vi "Register Sessions Impl.vi"(8 "error in":errorcluster, 11 "data in":T1) -> (0 "error out":errorcluster, 3 "data out":T1)   [LabVIEW 2020, in "MeasurementLink Session Management.lvlib" / "Session Reservation.lvclass"]
uses:
  Session Reservation.lvclass
  Data.ctl
  Connection Map/Connection Map.lvclass
  IState/IState.lvclass
  Session and Driver Info.ctl
  MeasurementLink Instrument/IInstrument/IInstrument.lvclass
  MeasurementLink Session Management Client/RPC Messages/ni_measurementlink_sessionmanagement_v1_SessionInformation.ctl
  MeasurementLink Session Management Client/RPC Messages/nidevice_grpc_Session.ctl
  MeasurementLink Session Management Client/RPC Messages/ni_measurementlink_sessionmanagement_v1_ChannelMapping.ctl
  MeasurementLink Session Management Client/RPC Messages/ni_measurementlink_PinMapContext.ctl
  MeasurementLink gRPC Utilities/gRPC Client Pool/FGV Action.ctl
  MeasurementLink Session Management Client/RPC Messages/ni_measurementlink_sessionmanagement_v1_RegisterSessionsRequest.ctl
  MeasurementLink gRPC Utilities/gRPC Client Pool/gRPC Client Pool.lvclass
  MeasurementLink Session Management Client/MeasurementLink Session Management Client.lvlib
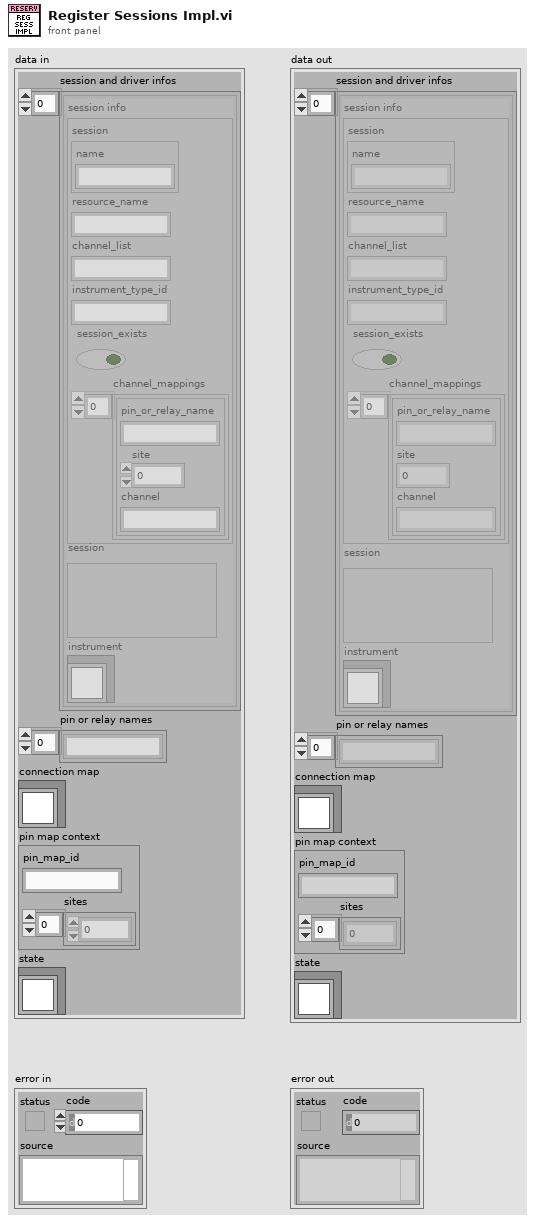
[diagram p1: front panel]
types:
  T1 = typedef "MeasurementLink Session Management.lvlib/Session Reservation.lvclass/Data.ctl" = cluster{"session and driver infos":T2[], "pin or relay names":string[], "connection map":refnum<class "Connection Map.lvclass">, "pin map context":T6, "state":refnum<class "IState.lvclass">}
  T2 = typedef "MeasurementLink Session Management.lvlib/Session Reservation.lvclass/Session and Driver Info.ctl" = cluster{"session info":T3, "session":variant, "instrument":refnum<class "IInstrument.lvclass">}
  T3 = typedef "MeasurementLink Session Management Client.lvlib/ni_measurementlink_sessionmanagement_v1_SessionInformation.ctl" = cluster{"session":T4, "resource_name":string, "channel_list":string, "instrument_type_id":string, "session_exists":bool, "channel_mappings":T5[]}
  T4 = typedef "MeasurementLink Session Management Client.lvlib/nidevice_grpc_Session.ctl" = cluster{"name":string}
  T5 = typedef "MeasurementLink Session Management Client.lvlib/ni_measurementlink_sessionmanagement_v1_ChannelMapping.ctl" = cluster{"pin_or_relay_name":string, "site":i32, "channel":string}
  T6 = typedef "MeasurementLink Session Management Client.lvlib/ni_measurementlink_PinMapContext.ctl" = cluster{"pin_map_id":string, "sites":i32[]}
  T7 = typedef "MeasurementLink Session Management Client.lvlib/ni_measurementlink_sessionmanagement_v1_RegisterSessionsRequest.ctl" = cluster{"sessions":T3[]}
  T8 = typedef "MeasurementLink gRPC Utilities.lvlib/gRPC Client Pool.lvclass/FGV Action.ctl" = enum16{"Get Discovery Client", "Get Session Client", "Get Pinmap Client", "Destroy Clients"}
  T9 = typedef "grpc-lvsupport-release.lvlib/grpcId.ctl" = u64
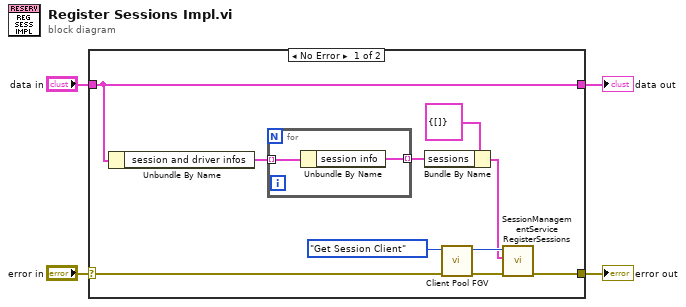
[diagram p0: block diagram]
diagram:
  n1 = case shown="No Error" "error in" {
    selector: "error in" -> [w6 w17]
    tunnel: "data in" -> [w7 w18]
    tunnel: [w7 w18] -> w2
    tunnel: [w5 w17] -> w1
    frame No Error {
      n2 = Unbundle By Name(w7) -> ("session and driver infos"=w8:T2[])
      n3 = for {
        tunnel: w8 -> [w16] mode=indexing
        tunnel: [w15] -> w10 mode=indexing
        n4 = Unbundle By Name(w16) -> ("session info"=w15:T3)
      }
      n5 = Bundle By Name(cluster=T7 {"sessions"=[]} ("Request Data"), "sessions"=w10) -> (w9:T7)
      n6 = call "Client Pool FGV.vi"("error in (no error)"=w6, "Action"=FGV_Action."Get Session Client") -> ("error out"=w13:errorcluster, "grpc client id"=w12:T9)  [unwired: 8 in]
      n7 = call "SessionManagementService RegisterSessions.vi"("error in"=w13, "Request Data"=w9, "gRPC ID"=w12) -> ("error out"=w5:errorcluster)  [unwired: 6 in, 2 out]
    }
    frame Error {
    }
  }
  "error out" <- w1
  "data out" <- w2
